vi "MazeGameIdToMazeSiteId.vi"(5 "MazeID":T4) -> (2 "MazeSiteID":cluster{"RoomID":T1, "WallID":T2, "DoorID":T3})   [LabVIEW 2020, in "FactoryMethod.lvlib" / "ParameterizedFactoryMethod.lvlib" / "MazeGame.lvclass"]
uses:
  MazeGame.lvclass
  API/TypeDef/MazeGameID.ctl
  API/TypeDef/RoomID.ctl
  API/TypeDef/WallID.ctl
  API/TypeDef/DoorID.ctl
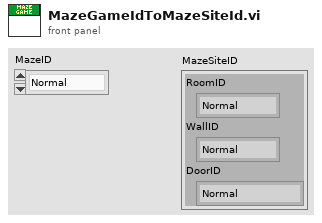
[diagram p1: front panel]
types:
  T1 = typedef "FactoryMethod.lvlib/ParameterizedFactoryMethod.lvlib/MazeGame.lvclass/RoomID.ctl" = enum16{"Normal", "Bombed", "Enchanted"}
  T2 = typedef "FactoryMethod.lvlib/ParameterizedFactoryMethod.lvlib/MazeGame.lvclass/WallID.ctl" = enum8{"Normal", "Bombed"}
  T3 = typedef "FactoryMethod.lvlib/ParameterizedFactoryMethod.lvlib/MazeGame.lvclass/DoorID.ctl" = enum8{"Normal", "Enchanted"}
  T4 = typedef "FactoryMethod.lvlib/ParameterizedFactoryMethod.lvlib/MazeGame.lvclass/MazeGameID.ctl" = enum16{"Normal", "Bombed", "Enchanted"}
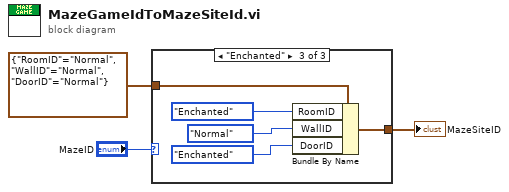
[diagram p0: block diagram]
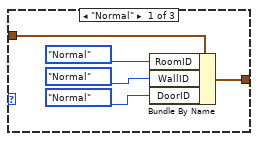
[diagram p2: hidden frame]
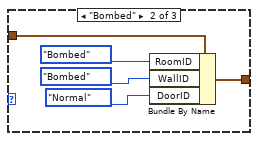
[diagram p3: hidden frame]
diagram:
  n1 = case shown="\"Enchanted\"" "MazeID" {
    tunnel: cluster{"RoomID":T1, "WallID":T2, "DoorID":T3} {"RoomID"=enum."Normal", "WallID"=enum."Normal", "DoorID"=enum."Normal"} ("MazeSiteID") -> [w8 w13 w18]
    tunnel: [w7 w12 w17] -> w1
    frame "Normal" {
      n2 = Bundle By Name(cluster=w8, "RoomID"=RoomID."Normal", "WallID"=WallID."Normal", "DoorID"=DoorID."Normal") -> (w7:cluster{"RoomID":T1, "WallID":T2, "DoorID":T3})
    }
    frame "Bombed" {
      n3 = Bundle By Name(cluster=w13, "RoomID"=RoomID."Bombed", "WallID"=WallID."Bombed", "DoorID"=DoorID."Normal") -> (w12:cluster{"RoomID":T1, "WallID":T2, "DoorID":T3})
    }
    frame "Enchanted" {
      n4 = Bundle By Name(cluster=w18, "RoomID"=RoomID."Enchanted", "WallID"=WallID."Normal", "DoorID"=DoorID."Enchanted") -> (w17:cluster{"RoomID":T1, "WallID":T2, "DoorID":T3})
    }
  }
  "MazeSiteID" <- w1
